vi "Secure-Release Region.vi"(6 "Test Run Number":dbl, 7 "Action":enum16{"Secure", "Release"}(ring), 8 "error in (no error)":errorcluster, 10 "Control In":T1={"I-O.lvclass"=refnum, "Gantry"=refnum, "Dispenser"="COM1"}, 11 "Fixture in":refnum<class "Fixture.lvclass">) -> (0 "error out":errorcluster, 1 "Position":i32, 2 "Control Out":T1={"I-O.lvclass"=refnum, "Gantry"=refnum, "Dispenser"="COM1"}, 3 "Fixture out":refnum<class "Fixture.lvclass">)   [LabVIEW 2021, in "Fixture.lvclass"]
uses:
  Fixture.lvclass
  Controller/Controllers.ctl
  Controller/I-O/I-O.lvclass
  C:/Program Files (x86)/Aerotech/A3200/LabVIEW/2010/Bin/Aerotech.A3200.dll
  Program Files (x86)/Aerotech/A3200/LabVIEW/2010/Bin/Aerotech.A3200.dll
  Fixture.lvclass/Fixture.ctl
  Controller/Controller.lvclass
panel:
  out "Test Run Number 2":dbl
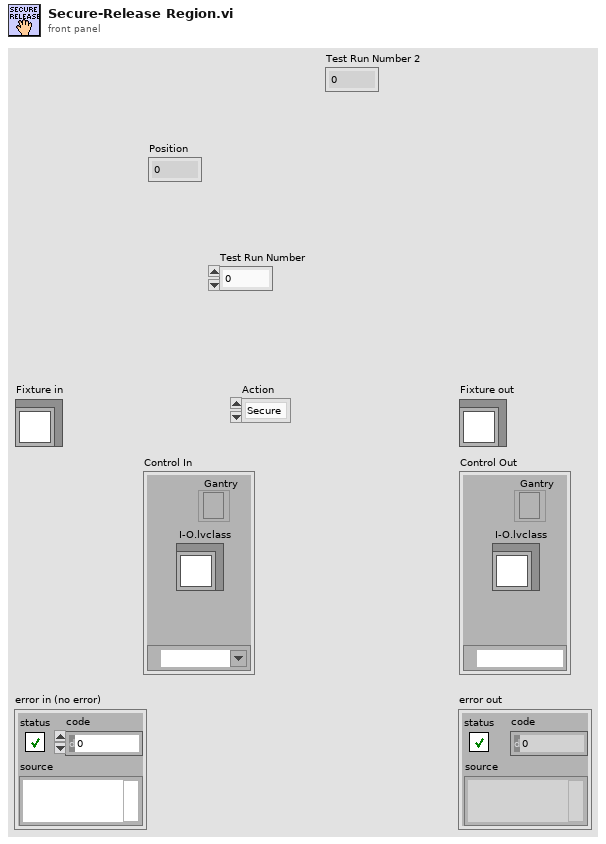
[diagram p1: front panel]
types:
  T1 = typedef "Controller.lvclass/Controllers.ctl" = cluster{"I-O.lvclass":refnum<class "I-O.lvclass">, "Gantry":refnum<k24>, "Dispenser":refnum<visa-resource-name>}
  T2 = typedef "I-O.lvclass/Pin Map.ctl" = cluster{"Region Valves":i32[], "Extra Valves":dbl[][][], "Tool Primary Valve":i32, "Tool Secondary Valve":i32, "Region Sensors":i32[], "Extra Sensors":dbl[][][], "Tool Primary Sensor":dbl, "Tool Secondary Sensor":dbl, "Compression Sensor":dbl, "5V":i32, "Dispenser Sensor":dbl, "Light Curtain":i32}
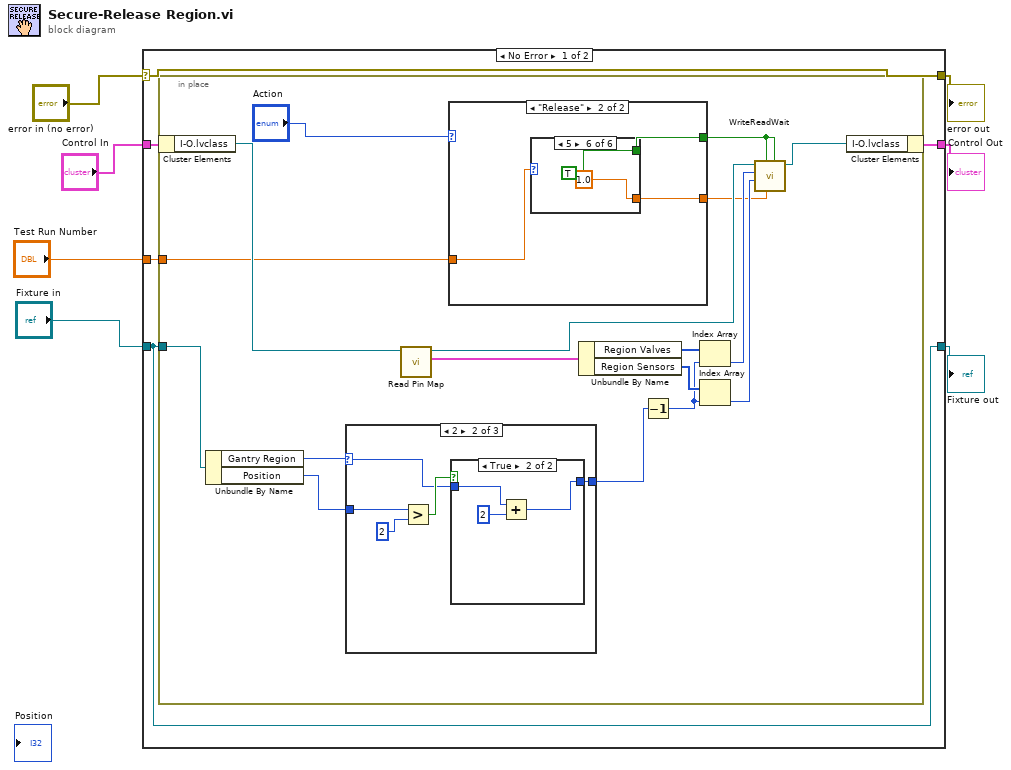
[diagram p0: block diagram]
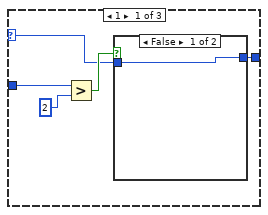
[diagram p2: hidden frame]
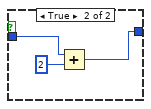
[diagram p3: hidden frame]
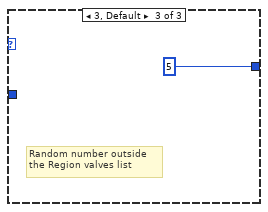
[diagram p5: hidden frame]
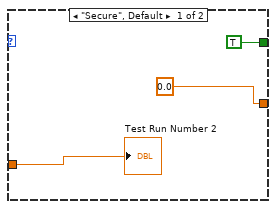
[diagram p6: hidden frame]
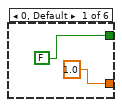
[diagram p7: hidden frame]
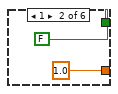
[diagram p8: hidden frame]
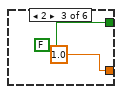
[diagram p9: hidden frame]
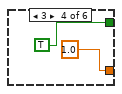
[diagram p10: hidden frame]
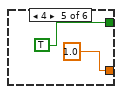
[diagram p11: hidden frame]
diagram:
  n1 = case shown="No Error" "error in (no error)" {
    selector: "error in (no error)" -> [w12 w69]
    tunnel: [w12 w69] -> w6
    tunnel: [w10 w68] -> w4
    tunnel: "Fixture in" -> [w10 w68]
    tunnel: "Control In" -> [w11 w67]
    tunnel: [w9 w67] -> w2
    tunnel: "Test Run Number" -> [w8 _]
    frame No Error {
      n2 = in-place {
        in-place-border: w10 -> [w28]
        in-place-border: w8 -> [w17]
        n3 = in-place-cluster #1(w11) -> ("I-O.lvclass"=w25:refnum<class "I-O.lvclass">)
        n4 = Unbundle By Name(w28) -> ("Gantry Region"=w15:i32, "Position"=w14:i32)
        n5 = case shown="2" w15 {
          selector: w15 -> [w30 w40 _]
          tunnel: [w33 w42 5] -> w16
          tunnel: w14 -> [w31 w39 _]
          frame 1 {
            n6 = Greater?(x=w31, y=2) -> (0:w32:bool)
            n7 = case shown="False" w32 {
              tunnel: w30 -> [w35 w37]
              tunnel: [w35 w36] -> w33
              frame False {
              }
              frame True {
                n8 = Add(x=w37, y=u32 2) -> (x+y=w36:u32)
              }
            }
          }
          frame 2 {
            n9 = Greater?(x=w39, y=2) -> (0:w41:bool)
            n10 = case shown="True" w41 {
              tunnel: w40 -> [w44 w46]
              tunnel: [w44 w45] -> w42
              frame False {
              }
              frame True {
                n11 = Add(x=w46, y=u32 2) -> (x+y=w45:u32)
              }
            }
          }
          frame 3, Default {
            # "Random number outside\nthe Region valves list"
          }
        }
        n12 = call-dynamic "Read Pin Map.vi"("I-O in"=w25) -> ("Pin Map 2"=w24:T2, "I-O out"=w23:refnum<class "I-O.lvclass">)  [unwired: 8 in, 1 out]
        n13 = case shown="\"Release\"" "Action" {
          tunnel: [TRUE w54] -> w26
          tunnel: w17 -> [w50 w53]
          tunnel: [0.0 w52] -> w13
          frame "Secure", Default {
            "Test Run Number 2" <- w50
          }
          frame "Release" {
            n14 = case shown="5" w53 {
              tunnel: [FALSE FALSE FALSE TRUE TRUE TRUE] -> w54
              tunnel: [1.0 1.0 1.0 1.0 1.0 1.0] -> w52
              frame 0, Default {
              }
              frame 1 {
              }
              frame 2 {
              }
              frame 3 {
              }
              frame 4 {
              }
              frame 5 {
              }
            }
          }
        }
        n15 = Unbundle By Name(w24) -> ("Region Valves"=w22:i32[], "Region Sensors"=w21:i32[])
        n16 = Decrement(x=w16) -> (x-1=w18:u32)
        n17 = Index Array(array=w22, index=w18) -> (element=w20:i32)
        n18 = Index Array(array=w21, index=w18) -> (element=w19:i32)
        n19 = call "WriteReadWait.vi"("Read Value"=w26, "Numeric"=w13, "Write Value"=w26, "Read"=w19, "Write"=w20, "I-O in"=w23) -> ("I-O out"=w29:refnum<class "I-O.lvclass">)  [unwired: 4 in, 1 out]
        n20 = in-place-cluster #1("I-O.lvclass"=w29) -> (w9:T1)
      }
    }
    frame Error {
    }
  }
  "error out" <- w6
  "Fixture out" <- w4
  "Control Out" <- w2
